vi "PumpMode Is Water.vi"(10 "PumpMode-Cluster out":T3(array[cluster]) {"concentratio mode" items=["water", "reagent"]; "Reagent" items=["HCl", "HF", "NH3", "HG", "PPM", "ORGANIC"]}, 11 "Numerisch":i32) -> (3 "is Water":bool)   [LabVIEW 2020, in "Linearisierung v2.lvlib" / "Gasteiler.lvlib" / "HovaCAL_Interface.lvlib" / "Helper.lvlib"]
uses:
  Controls/Pump Concentration Mode.ctl
  Controls/Reagent.ctl
  Helper.lvlib
  Controls/Controls.lvlib
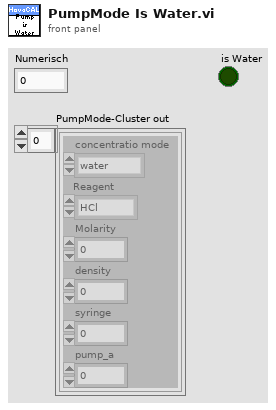
[diagram p1: front panel]
types:
  T1 = typedef "Linearisierung v2.lvlib/Gasteiler.lvlib/HovaCAL_Interface.lvlib/Controls.lvlib/Pump Concentration Mode.ctl" = i32
  T2 = typedef "Linearisierung v2.lvlib/Gasteiler.lvlib/HovaCAL_Interface.lvlib/Controls.lvlib/Reagent.ctl" = i32
  T3 = cluster{"concentratio mode":T1, "Reagent":T2, "Molarity":dbl, "density":dbl, "syringe":dbl, "pump_a":dbl}[]
  T4 = cluster{"concentratio mode":T1, "Reagent":T2, "Molarity":dbl, "density":dbl, "syringe":dbl, "pump_a":dbl}
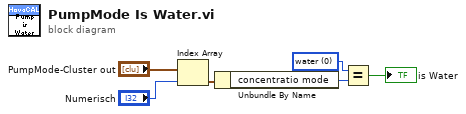
[diagram p0: block diagram]
diagram:
  w4 = T1 0 items=["water", "reagent"] ("x")
  n1 = Index Array(array="PumpMode-Cluster out", index="Numerisch") -> (element=w2:T4)
  n2 = Unbundle By Name(w2) -> ("concentratio mode"=w3:T1)
  n3 = Equal?(x=w4, y=w3) -> (x = y?=→"is Water":bool)
